vi "3.labtask2.vi"() -> ()   [LabVIEW 2022 SP3]
panel:
  out "x-y":u32
  out "Sampling period (ms)":dbl
  out "Total number of samples":dbl
  in  "Sampling rate (Hz)":dbl
  in  "Total duration (s)":dbl
  out "Waveform Graph":dynamicdata(graph)
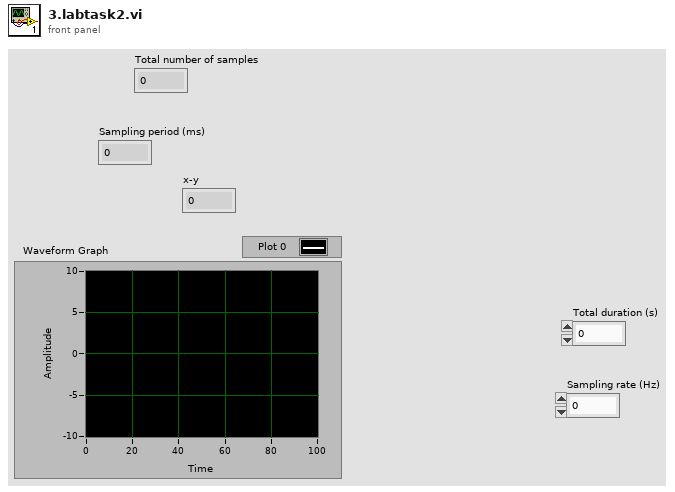
[diagram p1: front panel]
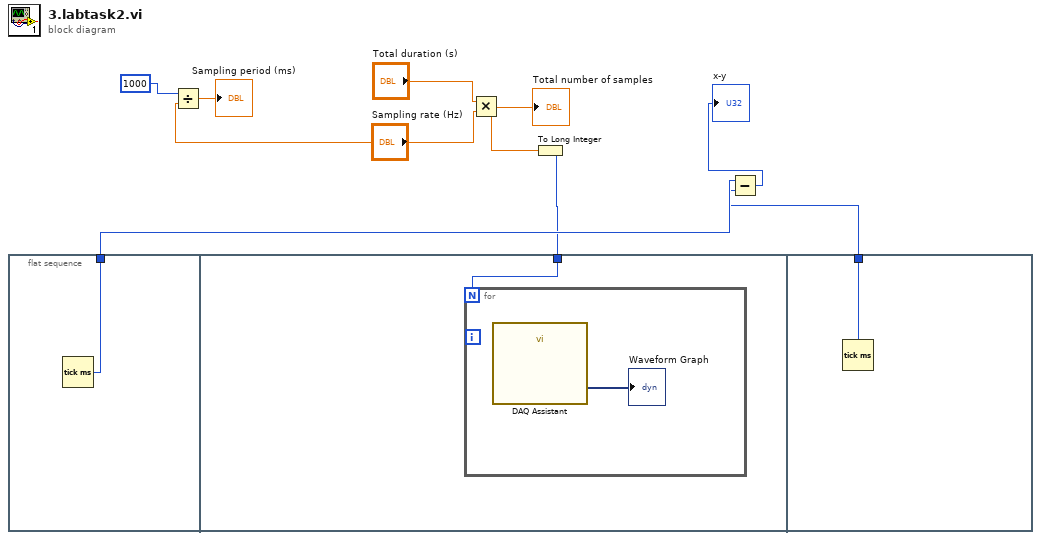
[diagram p0: block diagram]
diagram:
  n1 = flat-sequence {
    tunnel: [w10] -> w8
    tunnel: w1 -> [w11]
    tunnel: [w13] -> w7
    frame #0 {
      n2 = Tick Count (ms)() -> (millisecond timer value=w10:u32)
    }
    frame #1 {
      n3 = for {
        N: w11 -> [_]
        n4 = call "DAQ Assistant"() -> ("data"=→"Waveform Graph":dynamicdata)  [unwired: 17 in, 2 out]
      }
    }
    frame #2 {
      n5 = Tick Count (ms)() -> (millisecond timer value=w13:u32)
    }
  }
  n6 = Divide(x=1000, y="Sampling rate (Hz)") -> (x/y=→"Sampling period (ms)":dbl)
  n7 = Multiply(x="Total duration (s)", y="Sampling rate (Hz)") -> (x*y=w6:dbl)
  "Total number of samples" <- w6
  n8 = To Long Integer(number=w6) -> (32bit integer=w1:i32)
  n9 = Subtract(x=w8, y=w7) -> (x-y=→"x-y":u32)
